vi "ScanDelay_FTIR_LineScanSpectroscopy.vi"() -> ()   [LabVIEW 2022 SP3]
uses:
  Control_scanDelayWorkflow.ctl
  Control_GetSpectrum_LineScanSpectroscopy.ctl
panel:
  out "Line done":bool
  out "Data needed at new point":bool
  out "Sample Spectra at all accumulations":dbl[][][][](array[numeric])
  in  "Next Point":bool
  out "Current point\nindex":i32=1
  in  "# of spatial points":i32=2
  in  "Spectra view":enum32{"Point Spectrum", "Linescan Spectrum"}(tab)
  out "Normalized spectrum (amplitude)":T1(graph)
  out "Normalized spectrum (phase)":T1(graph)
  in  "Norm. smoothing":dbl=6.0 min=0.0 max=100.0 step=0.1
  in  "Flip anyway":bool
  out "Replicated wavelength (nm)":dbl=7692.0
  in  "Piecewise flattening":i16 min=0 max=10 step=1
  in  "Sample atten.\npowers (%)":dbl[](array[numeric])=[100.0, 100.0, 50.0, 50.0, 50.0, 50.0, 50.0, 50.0]
  in  "Sample power (%)":dbl(slide)=90.90909090909092 min=0.0 max=100.0 scale=0.0..100.0
  in  "Cyc. per intfg. (BB)":i32=30
  out "Attenuation factor":dbl=0.9090909090909092
  out "Replication wavelengths":dbl[](array[numeric])=[15300.0, 15300.0, 14800.0, 14800.0, 14500.0, 14500.0, 14100.0, 14100.0, 13700.0, 13333.0, 12500.0, 11765.0, 11111.0, 10526.0, 10000.0, 9524.0, 9091.0, 8696.0, 8333.0, 8000.0, 7692.0, 7407.0, 7143.0, 6897.0, 6667.0, 6452.0, 6250.0, 6061.0, 5882.0, 5714.0, 5556.0, 5405.0, 5263.0, 5000.0, 0.0]
  out "Replicator wavelengths loaded":bool=TRUE
  in  "Replic. path":path=path "C:/Users/mnopl/Desktop/Software/mnOPSuite/PRISM/Alpha replicator tables/2022.12.1 - 550-2000cm-1_x30_ExtraLowEnergyLiam.txt"
  in  "Load replic. table":bool
  in  "BB attenuation\npowers (%)":dbl[](array[numeric])=[100.0, 50.0, 2.0, 2.0, 2.0, 2.0, 2.0, 2.0]
  in  "Attenuation\nenergies (cm-1)":dbl[](array[numeric])=[500.0, 750.0, 1000.0, 1200.0, 1550.0, 1650.0, 1800.0, 2000.0]
  in  "BB power (%)":dbl(slide)=96.96969696969697 min=0.0 max=100.0 scale=0.0..100.0
  in  "Power threshold":dbl(slide)=343.04692863149205 scale=10.0..1000.0
  in  "Update alignment":bool
  in  "Bright beam: alignment delay":i32=-12
  in  "Norm. phase offset":dbl
  in  "Bright beam: physical channels (inputV, ScanDelay X)":tag="Dev1/ai2,Dev1/ai3"
  in  "Sample: physical channels (inputV, ScanDelay X)":tag="Dev1/ai2,Dev1/ai3"
  in  "Sample: alignment delay":i32=-12
  in  "Path to save\nnormalized spectrum":path=path "D:/Dropbox/Data/Park-SNOM/2022.07.19 - Liam - Strained STO/12_7 Measurements/STO_NormTo_Au_S2.txt"
  in  "Save normalized\nspectrum":bool
  in  "Optimize\ninterferogram\nalignment":bool
  in  "Toggle BB\nmirror\nUp / Down":bool=TRUE
  in  "Realign phase":bool=TRUE
  in  "Level phase":bool=TRUE
  in  "Pause\nacquisition":bool
  in  "Replicate\nfrom #":i8 min=0
  in  "Envelope width":dbl(slide)=1.6893939393939394 scale=0.25..4.0
  in  "BB-reference spectrum":bool
  in  "Acquire only\nBB 100% curve":bool=TRUE
  in  "Toggle pause (ms)":dbl=1000.0
  out "BB-referenced spectrum (phase)":T1(graph)
  out "BB-referenced spectrum (amplitude)":T2(graph)
  out "Reference BB spectra":dbl[][](array[numeric])
  out "Reference spectra":dbl[][](array[numeric])
  out "Latest alpha cmd":string="@mir setpump 90.9"
  in  "Replicate\nalpha on\naccumulation":bool
  out "# Accumulated":i32=2
  in  "# of Accumulations":i32=2
  in  "Cancel\nacquisition":bool
  out "Toggle position":i32=2
  out "Spectrum stored":bool=TRUE
  out "Reference stored":bool
  in  "Store as reference":bool
  out "Python alpha rep path":path=path "C:/Users/mnopl/Desktop/software/mnOPSuite/PRISM/python/alpha.py"
  out "Activity status":string="Awaiting command"
  out "Acquisition status":string="Ready to acquire spectrum"
  in  "Path to save spectrum":path=path "D:/Dropbox/Data/Park-SNOM/2022.07.19 - Liam - Strained STO/11_30 Measurements/Spectra/S2_AuRef12_9.txt"
  in  "Load reference":bool
  in  "Path to load reference":path=path "D:/Dropbox/Data/Park-SNOM/2022.07.19 - Liam - Strained STO/12_7 Measurements/STO_undeformed_S2.txt"
  in  "Path to load spectrum":path=path "D:/Dropbox/Data/Park-SNOM/2022.07.19 - Liam - Strained STO/12_7 Measurements/STO_undeformed_S2.txt"
  in  "Apply spectral\nenvelope":bool=TRUE
  out "Binned interferogram":cluster{"X":dbl, "Y":dbl}[](graph)
  out "Sample BB Spectra":dbl[][](array[numeric])
  out "Python error: spectrum acquisition":errorcluster
  out "Python scandelay path":path=path "C:/Users/mnopl/Desktop/software/mnOPSuite/PRISM/python/scandelay_FTIR.py"
  in  "Time per\nacquisition (s)":dbl=0.18
  in  "Sampling rate":dbl=250000.0
  in  "Delay calibratior\nfactor (ps/V)":dbl=-2.432 format="%_6g"
  in  "Cyc. / intfg.\n(sample)":i32=30
  out "Accumulated spectrum (amplitude)":T1(graph)
  out "Acquisition cycle":dbl[][](graph)
  out "% averaged":dbl=100.0
  in  "Halt program":bool=TRUE
  out "Python error: activity loop":errorcluster
  in  "Load spectrum":bool
  in  "Save spectrum":bool
  in  "Normalize spectrum":bool
  in  "Acquire spectrum":bool
  # "ai6 (7ps): -2 to -5"
  # "ai2 (7ps): -12 to -15"
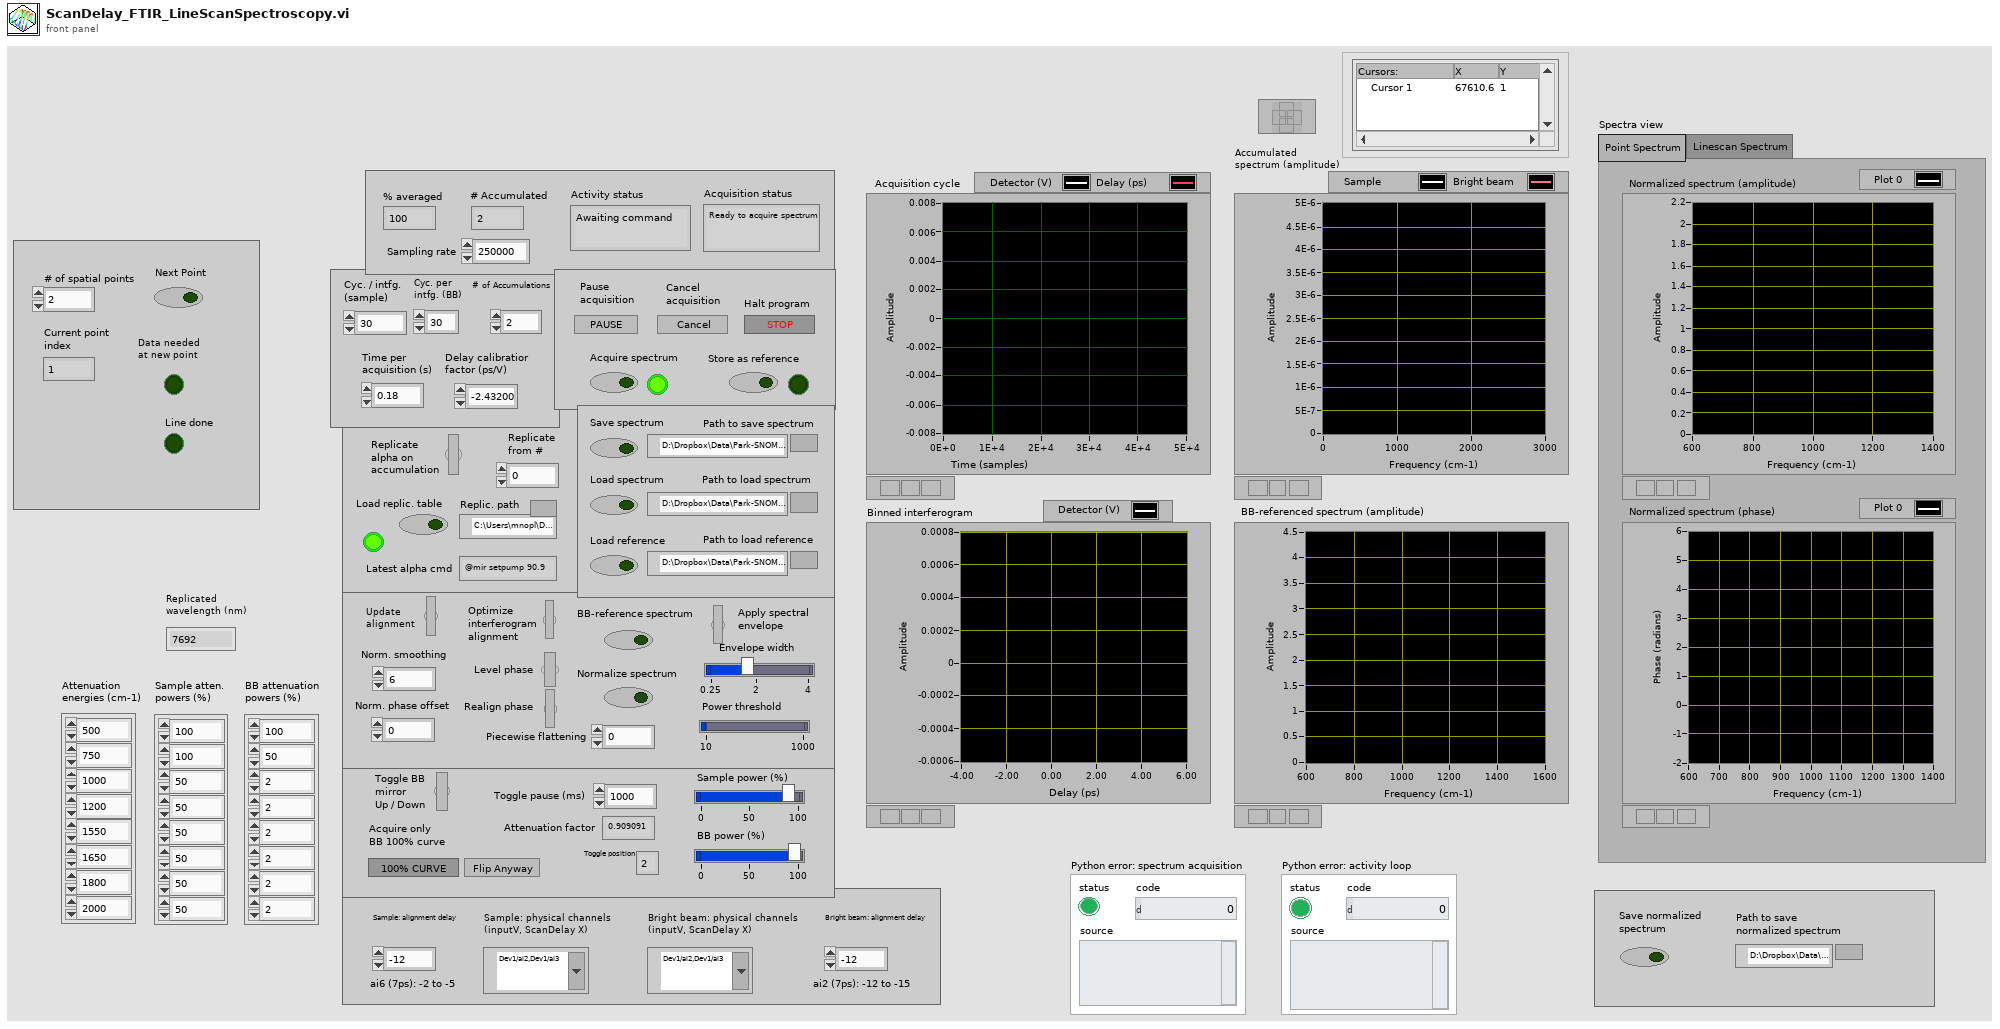
[diagram p1: front panel]
types:
  T1 = cluster{"Output spectrum":dbl[], "Output spectrum":dbl[]}
  T2 = cluster{"Sample Spectra":dbl[], "Sample Spectra":dbl[]}
  T3 = typedef "Control_scanDelayWorkflow.ctl" = enum16{"Initialize", "Sit Idle", "Load replicator table", "Flip BB", "Load Spectrum", "Store reference", "Save Spectrum", "Load reference", "Check Reference", "Check Spectrum", "BB reference spectrum", "Normalize Spectrum", "Save normalized spectrum", "Done"}
  T4 = typedef "imagedata.ctl" = cluster{"image type":i32, "image depth":i32, "image":u8[], "mask":u8[], "colors":u32[], "Rectangle":cluster{"left":i16, "top":i16, "right":i16, "bottom":i16}}
  T5 = typedef "Control_GetSpectrum_LineScanSpectroscopy.ctl" = enum16{"Initialize", "Replicate alpha", "Flip in BB", "Attenuate alpha", "Get Spectrum", "Accumulate BB spectrum", "Flip out BB", "Accumulate sample spectrum", "Await next point", "Assess accumulation", "Finalize", "Done"}
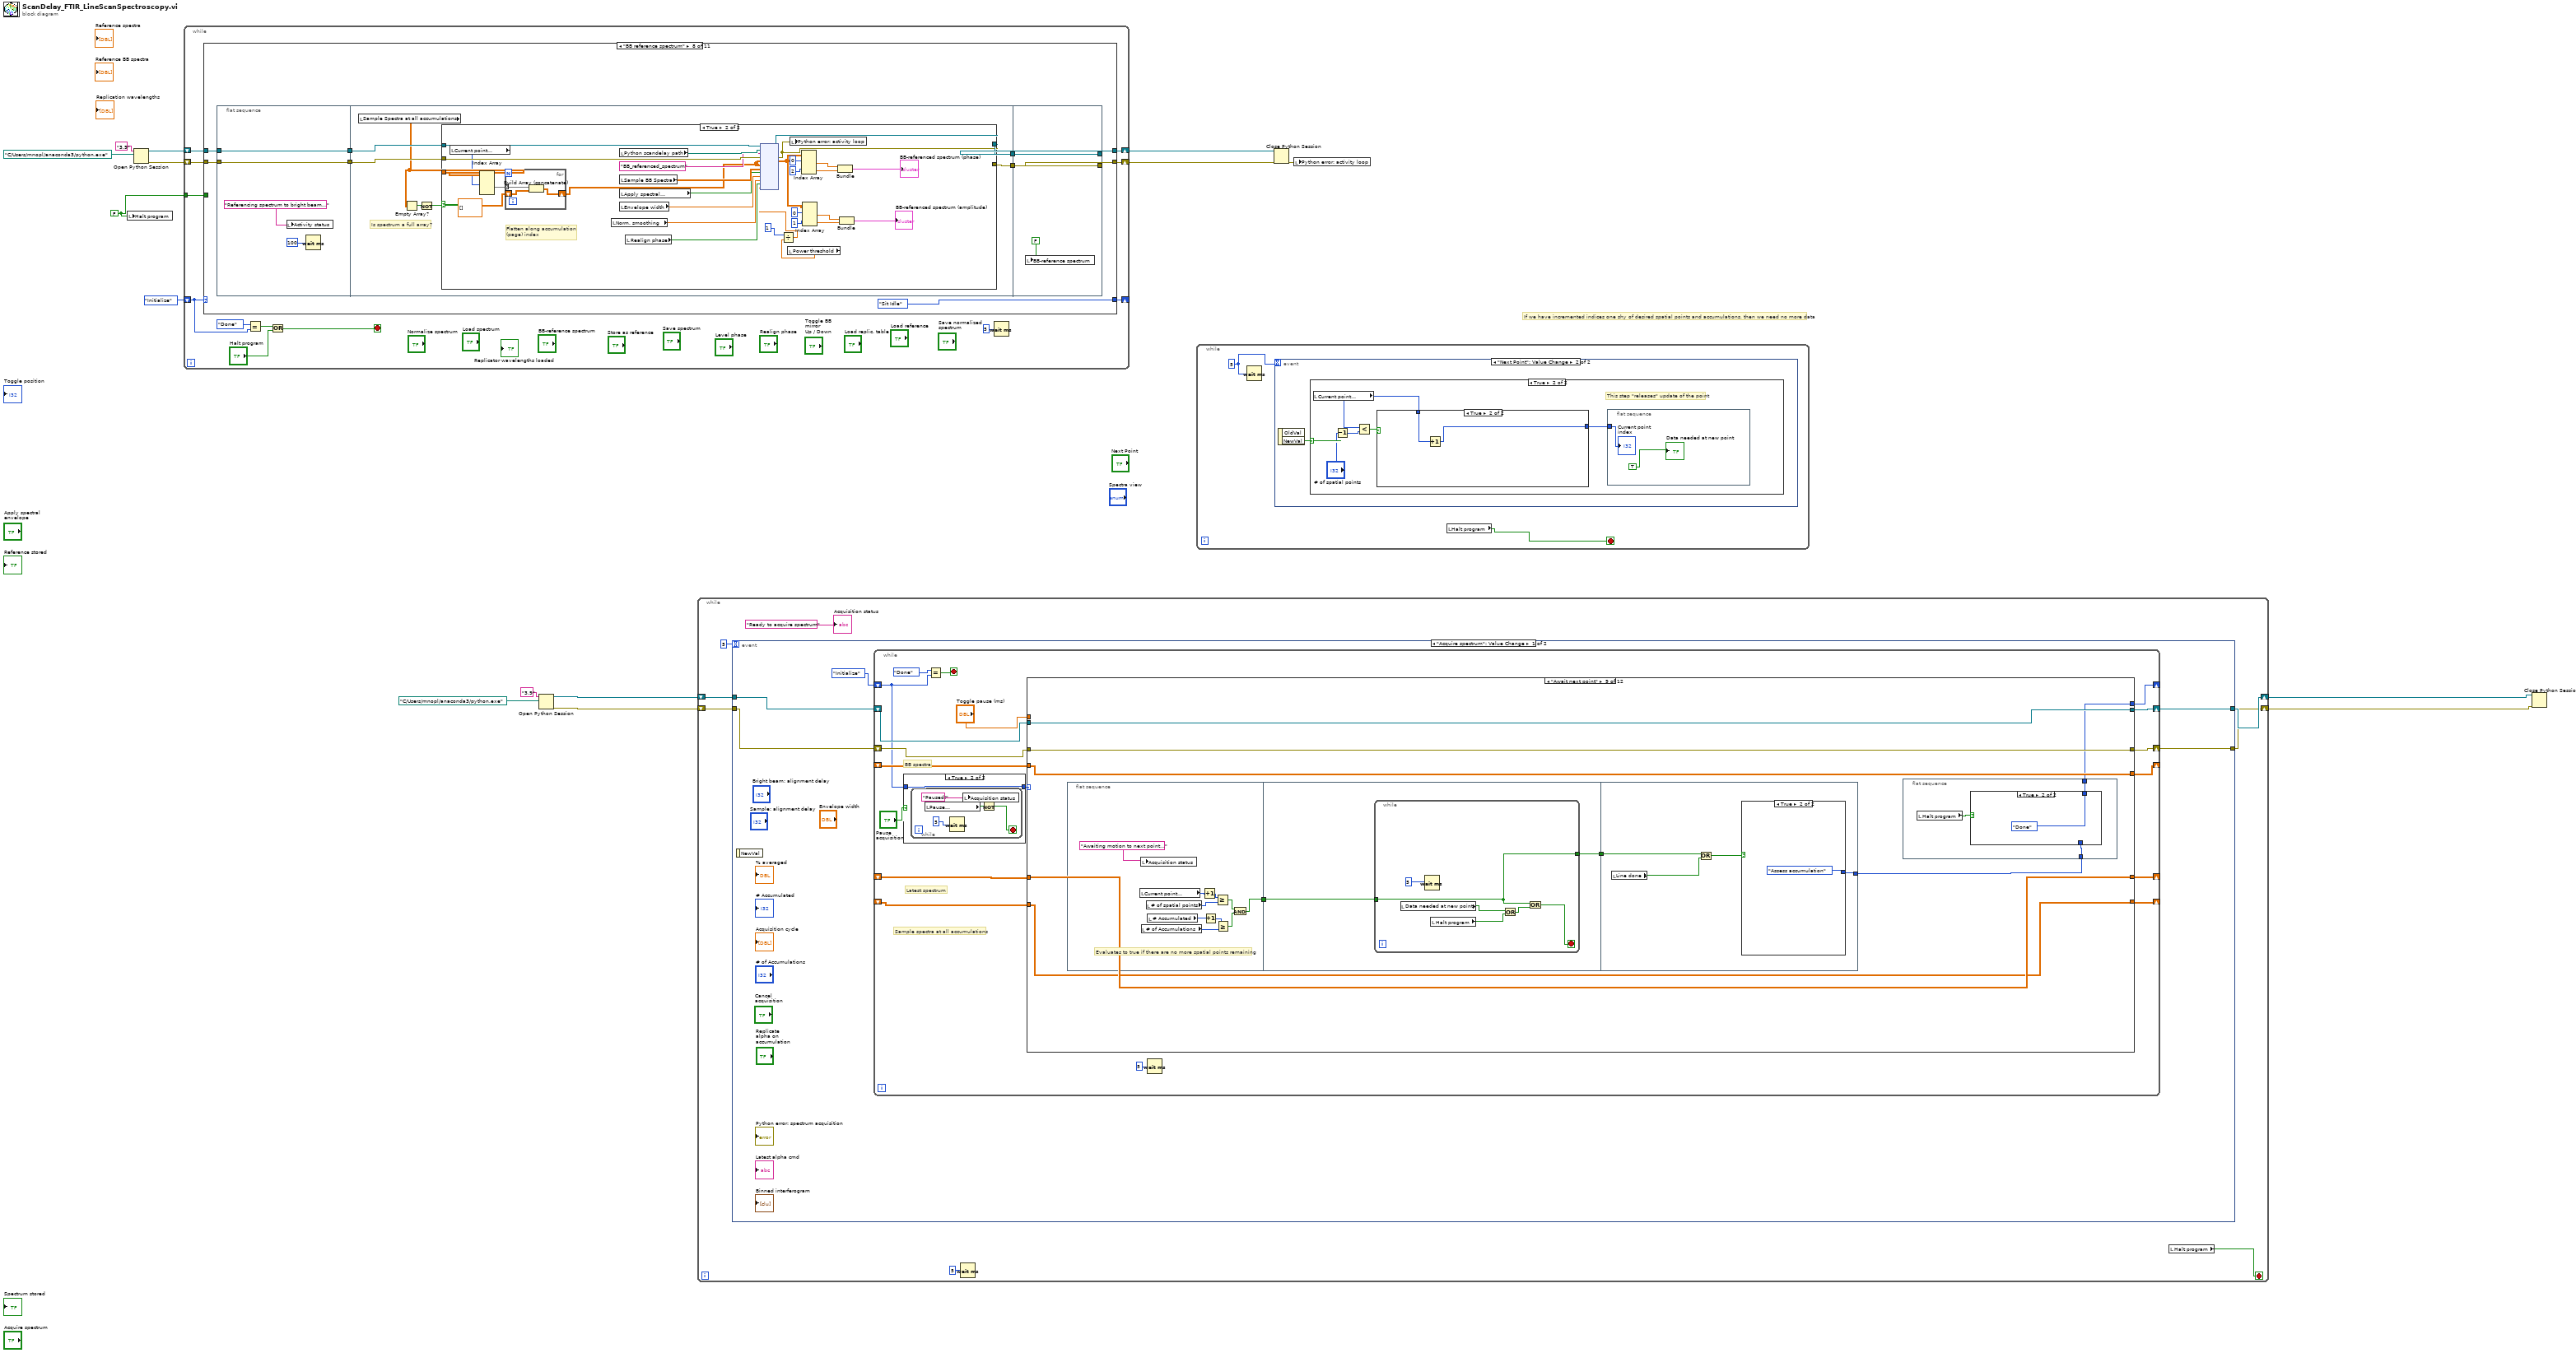
[diagram p0: block diagram]
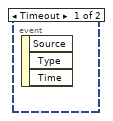
[diagram p2: hidden frame]
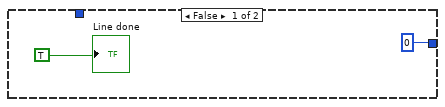
[diagram p4: hidden frame]
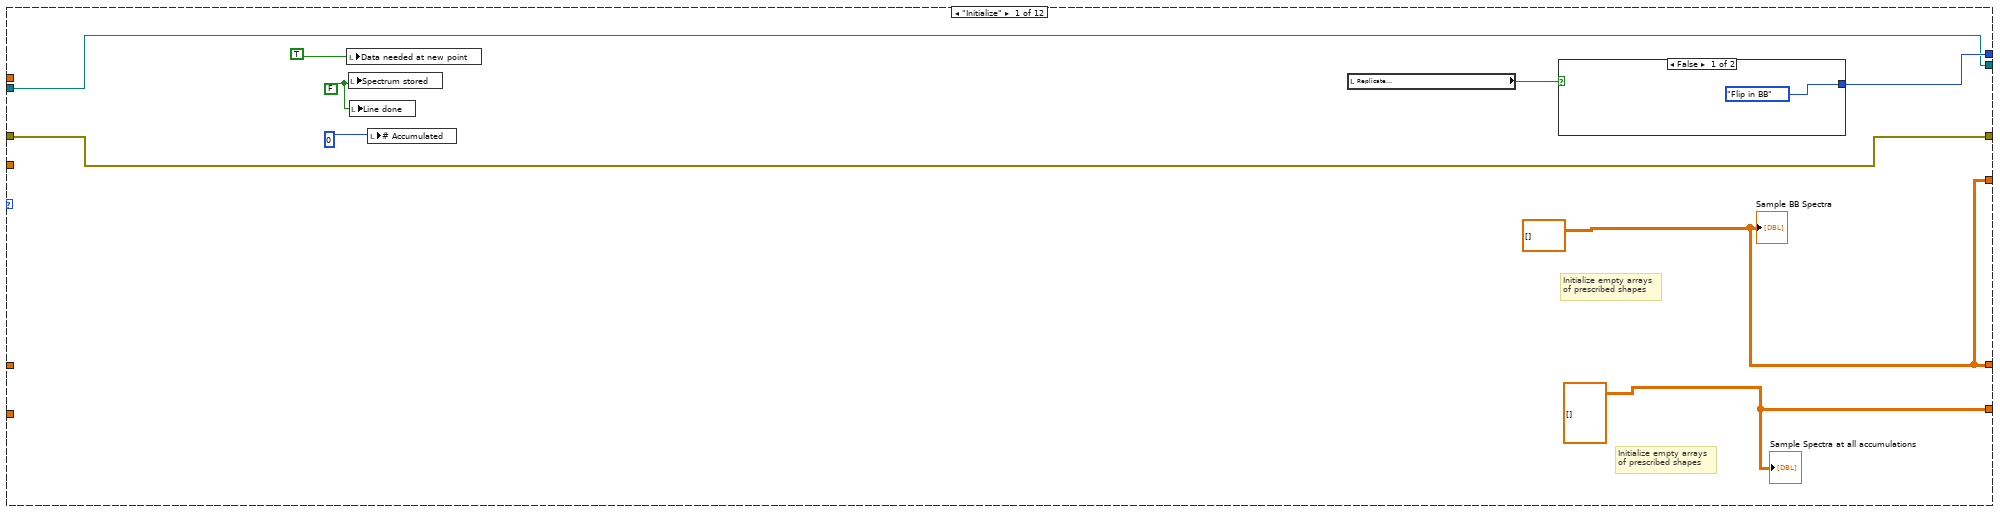
[diagram p6: hidden frame]
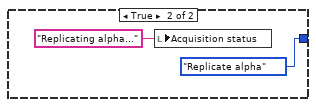
[diagram p7: hidden frame]
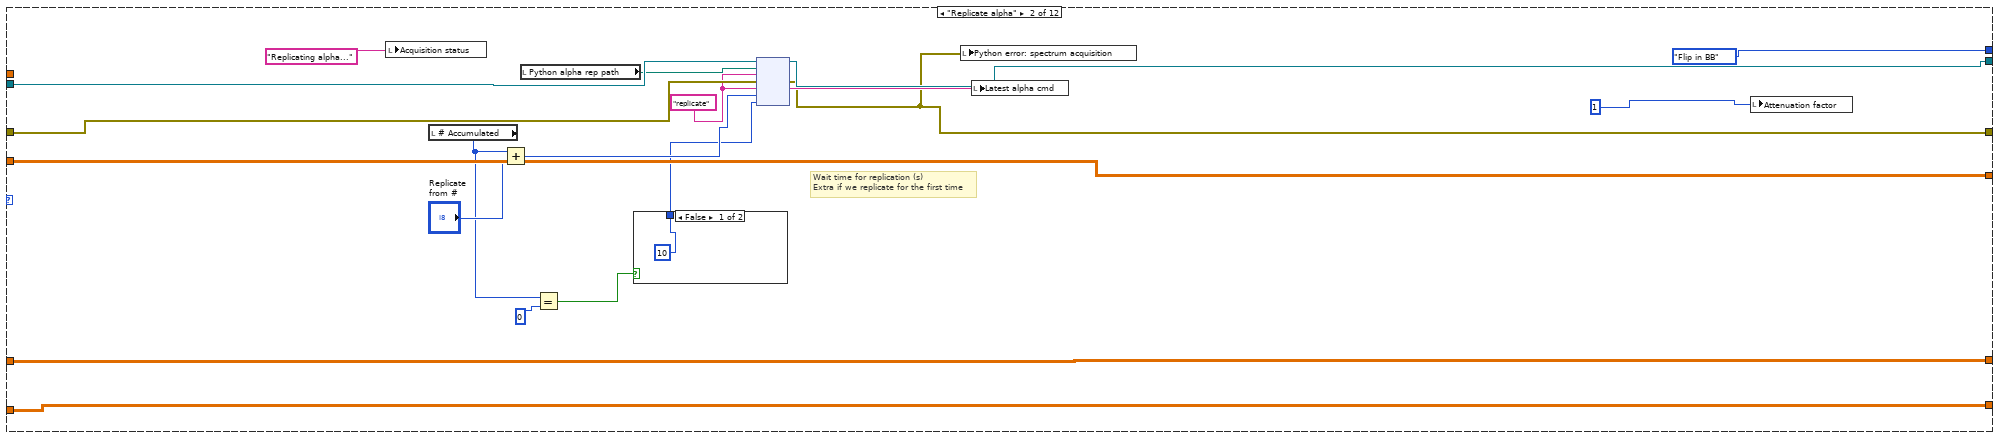
[diagram p8: hidden frame]
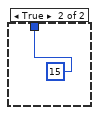
[diagram p9: hidden frame]
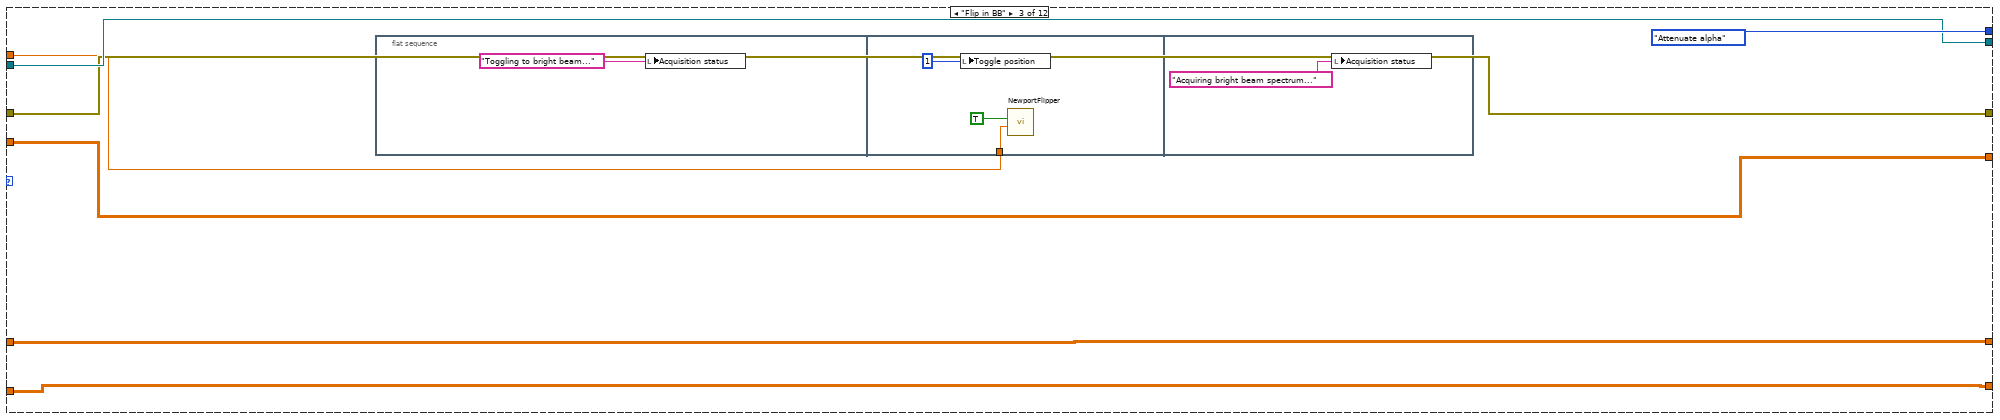
[diagram p10: hidden frame]
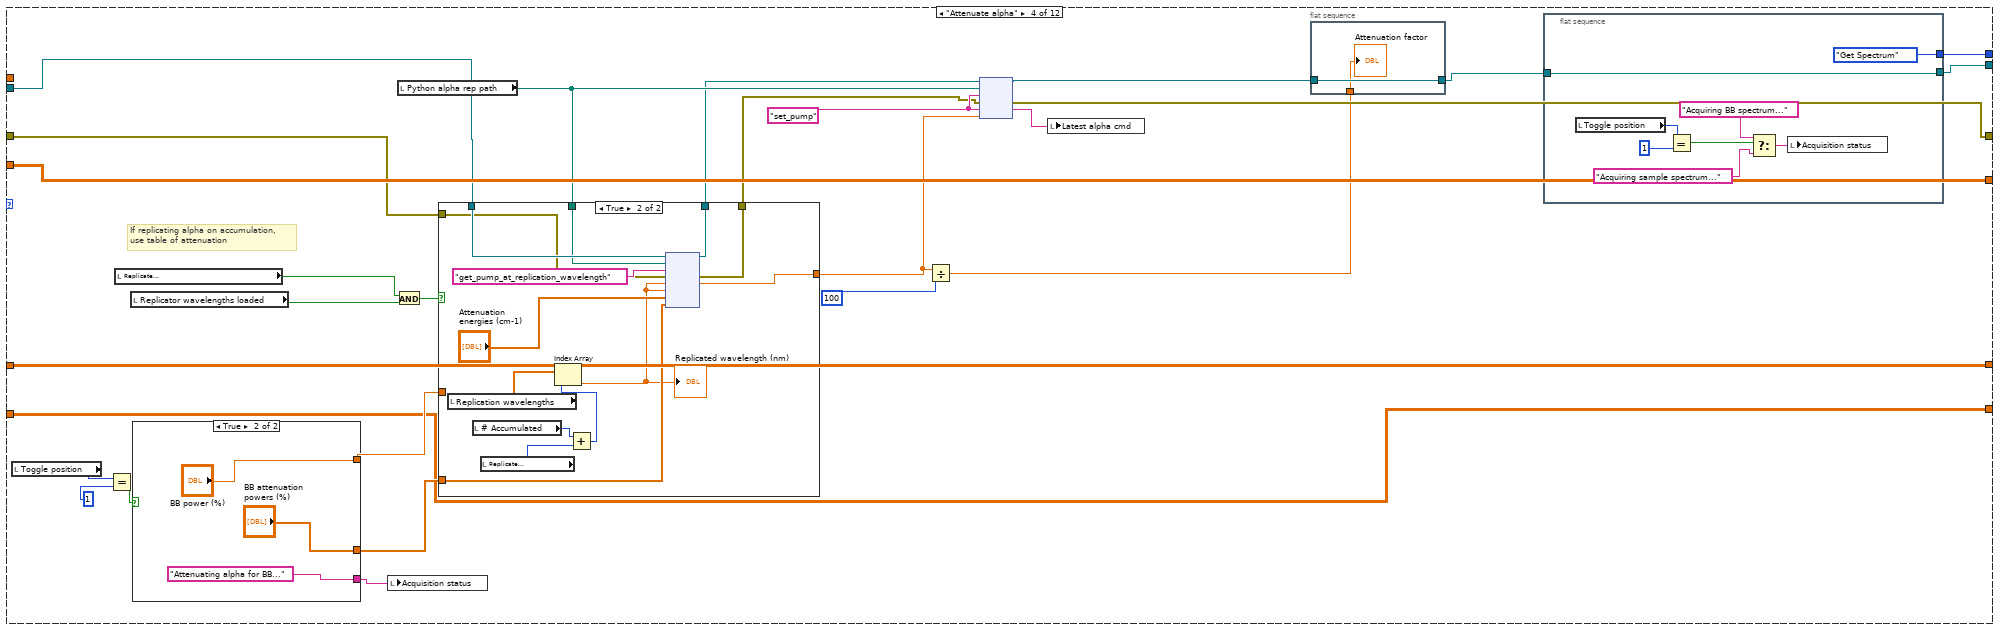
[diagram p11: hidden frame]
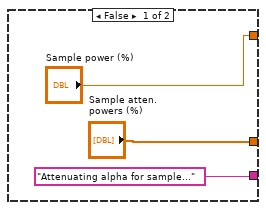
[diagram p12: hidden frame]
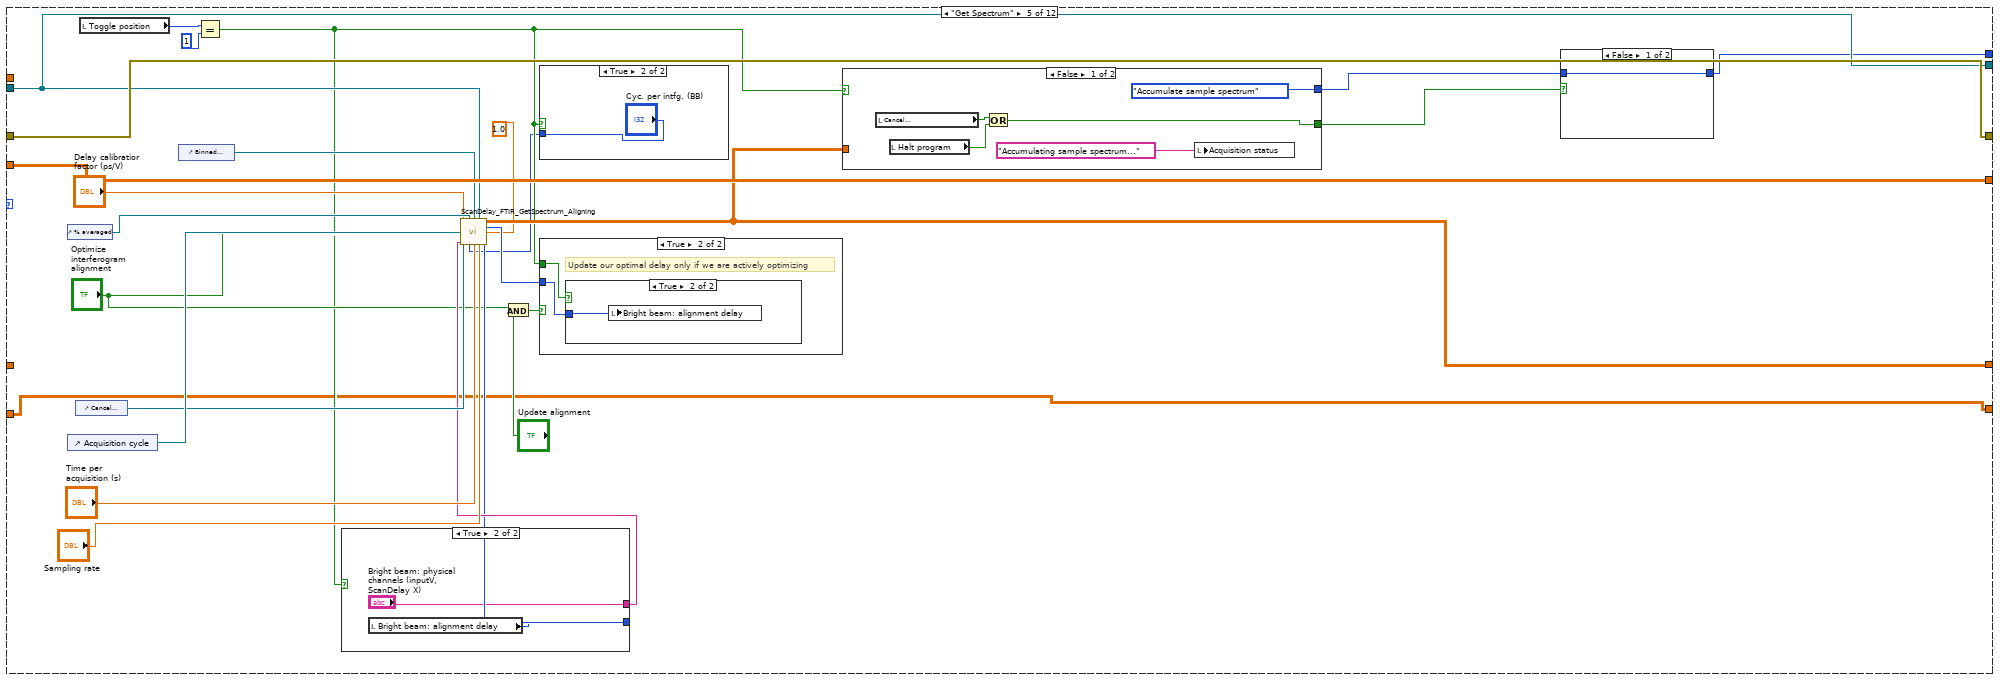
[diagram p14: hidden frame]
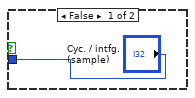
[diagram p15: hidden frame]
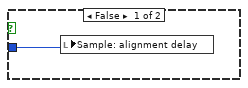
[diagram p17: hidden frame]
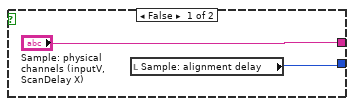
[diagram p18: hidden frame]
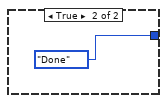
[diagram p19: hidden frame]
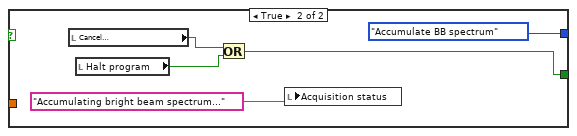
[diagram p20: hidden frame]
diagram:
  w1 = FALSE
  # "If we have incremented indices one shy of desired spatial points and accumulations, then we need no more data"
  n1 = local write "Halt program"(w1) -> ()
  n2 = Open Python Session(python version="3.9", python path=path "C:/Users/mnopl/anaconda3/python.exe") -> (session out=w11:refnum<k35>, error out=w10:errorcluster)  [unwired: 1 in]
  n3 = while {
    shift-right: [w20] -> _
    shift-left: Control_scanDelayWorkflow."Initialize" -> [w17]
    shift-right: [w26] -> w12
    shift-left: w10 -> [w18]
    shift-right: [w21] -> w13
    shift-left: w11 -> [w19]
    tunnel: w1 -> [w16]
    stop <- w24 stop-if-true
    n4 = case shown="\"BB reference spectrum\"" w17 {
      tunnel: [w31 w74 w93 w115 w136 w193 w216 w227 w280 w287 w331] -> w26
      tunnel: w19 -> [w32 w73 w92 w116 w139 w194 w217 w225 w281 w288 w332]
      tunnel: w18 -> [w31 w74 w93 w115 w138 w193 w216 w224 w280 w287 w331]
      tunnel: [w32 w73 w92 w116 w137 w194 w217 w226 w281 w288 w332] -> w21
      tunnel: [w30 Control_scanDelayWorkflow."Sit Idle" Control_scanDelayWorkflow."Sit Idle" Control_scanDelayWorkflow."Sit Idle" Control_scanDelayWorkflow."Sit Idle" Control_scanDelayWorkflow."Sit Idle" Control_scanDelayWorkflow."Sit Idle" Control_scanDelayWorkflow."Sit Idle" Control_scanDelayWorkflow."Sit Idle" Control_scanDelayWorkflow."Sit Idle" Control_scanDelayWorkflow."Sit Idle"] -> w20
      tunnel: w16 -> [_ _ _ _ _ _ w213 _ _ _ _]
      frame "Sit Idle", Default {
        n5 = event shown="[9] Timeout" {
          selector: _ -> [_ _ _ _ _ _ _ _ _ _]
          dyn-events: _ -> [_ _ _ _ _ _ _ _ _ _]
          timeout: 5 -> [_ _ _ _ _ _ _ _ _ w66]
          tunnel: [w33 w37 w44 Control_scanDelayWorkflow."Flip BB" w46 w50 w54 w58 w62 Control_scanDelayWorkflow."Sit Idle"] -> w30
          event "Normalize spectrum": Value Change {
            n6 = event-data() -> ("NewVal"=w34:bool)  [unwired: 1 in]
            n7 = Select(t=Control_scanDelayWorkflow."Normalize Spectrum", s=w34, f=Control_scanDelayWorkflow."Sit Idle") -> (s? t:f=w33:T3)
          }
          event "Store as reference": Value Change {
            n8 = event-data() -> ("NewVal"=w40:bool)  [unwired: 1 in]
            n9 = Select(t=Control_scanDelayWorkflow."Store reference", s=w40, f=Control_scanDelayWorkflow."Sit Idle") -> (s? t:f=w37:T3)
          }
          event "BB-reference spectrum": Value Change {
            n10 = event-data() -> ("NewVal"=w42:bool)  [unwired: 1 in]
            n11 = Select(t=Control_scanDelayWorkflow."BB reference spectrum", s=w42, f=Control_scanDelayWorkflow."Sit Idle") -> (s? t:f=w44:T3)
          }
          event "Toggle BB\nmirror\nUp / Down": Value Change {
            n12 = event-data() -> ()  [unwired: 1 in, 1 out]
          }
          event "Save normalized\nspectrum": Value Change {
            n13 = event-data() -> ("NewVal"=w47:bool)  [unwired: 1 in]
            n14 = Select(t=Control_scanDelayWorkflow."Save normalized spectrum", s=w47, f=Control_scanDelayWorkflow."Sit Idle") -> (s? t:f=w46:T3)
          }
          event "Load replic. table": Value Change {
            n15 = event-data() -> ("NewVal"=w53:bool)  [unwired: 1 in]
            n16 = Select(t=Control_scanDelayWorkflow."Load replicator table", s=w53, f=Control_scanDelayWorkflow."Sit Idle") -> (s? t:f=w50:T3)
          }
          event "Save spectrum": Value Change {
            n17 = event-data() -> ("NewVal"=w55:bool)  [unwired: 1 in]
            n18 = Select(t=Control_scanDelayWorkflow."Save Spectrum", s=w55, f=Control_scanDelayWorkflow."Sit Idle") -> (s? t:f=w54:T3)
          }
          event "Load reference": Value Change {
            n19 = event-data() -> ("NewVal"=w61:bool)  [unwired: 1 in]
            n20 = Select(t=Control_scanDelayWorkflow."Load reference", s=w61, f=Control_scanDelayWorkflow."Sit Idle") -> (s? t:f=w58:T3)
          }
          event "Load spectrum": Value Change {
            n21 = event-data() -> ("NewVal"=w63:bool)  [unwired: 1 in]
            n22 = Select(t=Control_scanDelayWorkflow."Load Spectrum", s=w63, f=Control_scanDelayWorkflow."Sit Idle") -> (s? t:f=w62:T3)
          }
          event Timeout {
            n23 = event-data() -> ()  [unwired: 1 in, 2 out]
            n24 = Wait (ms)(milliseconds to wait=w66) -> ()  [unwired: 1 out]
          }
        }
        "Activity status" <- "Awaiting command"
      }
      frame "Store reference" {
        # "Is spectrum a full array?"
        n25 = local read "Sample Spectra at all accumulations"() -> (w69:dbl[][][][])
        n26 = local read "Sample BB Spectra"() -> (w68:dbl[][])
        n27 = Empty Array?(array=w69) -> (empty?=w71:bool)
        n28 = Not(x=w71) -> (.not. x?=w70:bool)
        n29 = case shown="True" w70 {
          tunnel: w69 -> [_ w79]
          tunnel: w68 -> [_ w81]
          frame False {
            n30 = Wait (ms)(milliseconds to wait=1000) -> ()  [unwired: 1 out]
            n31 = local write "Activity status"("Error: Spectrum is empty!") -> ()
          }
          frame True {
            # "Flatten along accumulation\n(page) index"
            n32 = local read "Current point\nindex"() -> (w77:i32)
            n33 = Index Array(array=w79, index (dim 1)=w77) -> (element=w80:dbl[][][])  [unwired: 3 in]
            n34 = for {
              tunnel: w80 -> [w87] mode=indexing
              shift-right: [w86] -> w78
              shift-left: _ -> [w85]
              n35 = Build Array (concatenate)(w87, w85) -> (w86:dbl[][])
            }
            n36 = local write "Reference BB spectra"(w81) -> ()
            n37 = local write "Reference spectra"(w78) -> ()
            n38 = local write "Reference stored"(TRUE) -> ()
            n39 = Wait (ms)(milliseconds to wait=1000) -> ()  [unwired: 1 out]
            n40 = local write "Activity status"("Storing reference!") -> ()
          }
        }
      }
      frame "Save Spectrum" {
        # "Is spectrum a full array?"
        n41 = local read "Sample Spectra at all accumulations"() -> (w89:dbl[][][][])
        n42 = Empty Array?(array=w89) -> (empty?=w90:bool)
        n43 = Not(x=w90) -> (.not. x?=w88:bool)
        n44 = case shown="True" w88 {
          tunnel: w89 -> [_ w96]
          frame False {
            n45 = flat-sequence {
              frame #0 {
                n46 = local write "Activity status"("Error:  Spectrum is empty, cannot save!") -> ()
              }
              frame #1 {
                n47 = Wait (ms)(milliseconds to wait=1000) -> ()  [unwired: 1 out]
              }
            }
          }
          frame True {
            n48 = flat-sequence {
              tunnel: w96 -> [w97]
              frame #0 {
                w103 = "%g"
                n49 = Path To String(path="Path to save spectrum") -> (string=w106:string)
                n50 = local read "Sample BB Spectra"() -> (w98:dbl[][])
                n51 = Search and Replace String(input string=w106, search string="(.txt)*$", replace string=".txt") -> (result string=w110:string)  [unwired: 5 in, 3 out]
                n52 = Search and Replace String(input string=w110, search string=".txt$", replace string="_BB.txt") -> (result string=w109:string)  [unwired: 5 in, 3 out]
                n53 = String To Path(string=w110) -> (path=w107:path)
                n54 = Array To Spreadsheet String(array=w97, 3:w103) -> (spreadsheet string=w104:string)  [unwired: 1 in]
                n55 = Array To Spreadsheet String(array=w98, 3:w103) -> (spreadsheet string=w111:string)  [unwired: 1 in]
                n56 = String To Path(string=w109) -> (path=w108:path)
                n57 = Write to Text File(file (use dialog)=w107, text=w104) -> ()  [unwired: 2 in, 3 out]
                n58 = Write to Text File(file (use dialog)=w108, text=w111) -> ()  [unwired: 2 in, 3 out]
              }
              frame #1 {
                n59 = local write "Activity status"("Successfully saved spectrum!") -> ()
                n60 = Wait (ms)(milliseconds to wait=1000) -> ()  [unwired: 1 out]
              }
            }
          }
        }
      }
      frame "Load reference" {
        n61 = flat-sequence {
          frame #0 {
            w121 = "%g"
            n62 = Path To String(path="Path to load reference") -> (string=w117:string)
            n63 = Search and Replace String(input string=w117, search string=".txt$", replace string="_BB.txt") -> (result string=w119:string)  [unwired: 5 in, 3 out]
            n64 = Read from Text File(file (use dialog)="Path to load reference") -> (text=w122:string)  [unwired: 3 in, 3 out]
            n65 = String To Path(string=w119) -> (path=w126:path)
            n66 = Spreadsheet String To Array(format string=w121, spreadsheet string=w122) -> (array=w123:dbl[][])  [unwired: 2 in]
            n67 = Read from Text File(file (use dialog)=w126) -> (text=w125:string)  [unwired: 3 in, 3 out]
            n68 = local write "Reference spectra"(w123) -> ()
            n69 = Spreadsheet String To Array(format string=w121, spreadsheet string=w125) -> (array=w127:dbl[][])  [unwired: 2 in]
            n70 = local write "Reference BB spectra"(w127) -> ()
          }
          frame #1 {
            n71 = local write "Reference stored"(TRUE) -> ()
            n72 = Wait (ms)(milliseconds to wait=1000) -> ()  [unwired: 1 out]
            n73 = local write "Activity status"("Successfully loaded reference!") -> ()
          }
        }
      }
      frame "Normalize Spectrum" {
        n74 = local read "Reference stored"() -> (w133:bool)
        n75 = local read "Spectrum stored"() -> (w132:bool)
        n76 = And(x=w132, y=w133) -> (x .and. y?=w131:bool)
        n77 = flat-sequence {
          tunnel: w139 -> [w145]
          tunnel: w138 -> [w144]
          tunnel: [w143] -> w135
          tunnel: [w142] -> w134
          tunnel: w131 -> [w141]
          tunnel: [w190] -> w136
          tunnel: [w191] -> w137
          tunnel: w135 -> [w191]
          tunnel: w134 -> [w190]
          frame #0 {
            n78 = case shown="True" w141 {
              tunnel: w145 -> [w147 w184]
              tunnel: w144 -> [w146 w183]
              tunnel: [w147 w182] -> w143
              tunnel: [w146 w166] -> w142
              frame False {
                n79 = Wait (ms)(milliseconds to wait=1000) -> ()  [unwired: 1 out]
                n80 = local write "Activity status"("Error: Spectrum or reference is empty!") -> ()
              }
              frame True {
                # "Flatten along accumulation\n(page) index"
                n81 = local read "Sample Spectra at all accumulations"() -> (w152:dbl[][][][])
                n82 = local read "Current point\nindex"() -> (w151:i32)
                n83 = Index Array(array=w152, index (dim 1)=w151) -> (element=w153:dbl[][][])  [unwired: 3 in]
                n84 = for {
                  tunnel: w153 -> [w188] mode=indexing
                  shift-right: [w187] -> w150
                  shift-left: _ -> [w186]
                  n85 = Build Array (concatenate)(w188, w186) -> (w187:dbl[][])
                }
                n86 = Wait (ms)(milliseconds to wait=1000) -> ()  [unwired: 1 out]
                n87 = local read "Python scandelay path"() -> (w181:path)
                n88 = local read "Sample BB Spectra"() -> (w167:dbl[][])
                n89 = local read "Reference spectra"() -> (w165:dbl[][])
                n90 = local read "Reference BB spectra"() -> (w164:dbl[][])
                n91 = local read "Apply spectral\nenvelope"() -> (w163:bool)
                n92 = local read "Envelope width"() -> (w162:dbl)
                n93 = local read "Realign phase"() -> (w160:bool)
                n94 = local read "Level phase"() -> (w161:bool)
                n95 = local write "Activity status"("Normalizing spectrum!") -> ()
                n96 = Divide(x=1, y="Power threshold") -> (x/y=w155:dbl)
                n97 = node(w184, w181, "normalized_spectrum", w183, w150, w150, w167, w165, w164, w163, w162, w161, w160, "Norm. phase offset", "Norm. smoothing", w155, "Piecewise flattening") -> (w182:refnum<k35>, w166:errorcluster, w169:dbl[][])  [unwired: 12 in, 2 out]
                "Python error: activity loop" <- w166
                n98 = Index Array(array=w169, index (row) #1=0, index (row) #2=1) -> (element #1=w177:dbl[], element #2=w176:dbl[])  [unwired: 2 in]
                n99 = Index Array(array=w169, index (row) #1=0, index (row) #2=2) -> (element #1=w173:dbl[], element #2=w172:dbl[])  [unwired: 2 in]
                n100 = Bundle(w177, w176) -> (→"Normalized spectrum (amplitude)":cluster{dbl[], dbl[]})  [unwired: 1 in]
                n101 = Bundle(w173, w172) -> (→"Normalized spectrum (phase)":cluster{dbl[], dbl[]})  [unwired: 1 in]
              }
            }
          }
          frame #1 {
            n102 = local write "Normalize spectrum"(FALSE) -> ()
          }
        }
      }
      frame "Load Spectrum" {
        n103 = disable-structure shown="Disabled" {
          frame Disabled {
            n104 = flat-sequence {
              frame #0 {
                w202 = "%g"
                n105 = Path To String(path="Path to load spectrum") -> (string=w198:string)
                n106 = Search and Replace String(input string=w198, search string=".txt$", replace string="_BB.txt") -> (result string=w200:string)  [unwired: 5 in, 3 out]
                n107 = Read from Text File(file (use dialog)="Path to load spectrum") -> (text=w203:string)  [unwired: 3 in, 3 out]
                n108 = String To Path(string=w200) -> (path=w205:path)
                n109 = Spreadsheet String To Array(format string=w202, spreadsheet string=w203) -> (array=w196:dbl[][])  [unwired: 2 in]
                n110 = Read from Text File(file (use dialog)=w205) -> (text=w204:string)  [unwired: 3 in, 3 out]
                n111 = Spreadsheet String To Array(format string=w202, spreadsheet string=w204) -> (array=w195:dbl[][])  [unwired: 2 in]
                n112 = local write item#-1(w196) -> ()
                n113 = local write "Sample BB Spectra"(w195) -> ()
              }
              frame #1 {
                n114 = local write "Load spectrum"(FALSE) -> ()
                n115 = local write "Spectrum stored"(TRUE) -> ()
                n116 = local write "Activity status"("Successfully loaded spectrum!") -> ()
                n117 = Wait (ms)(milliseconds to wait=1000) -> ()  [unwired: 1 out]
              }
            }
          }
          frame Enabled {
          }
        }
      }
      frame "Initialize" {
        # "Fine so long as we've saved default values for \"replication wavelengths\""
        n118 = local write "Replicator wavelengths loaded"(TRUE) -> ()
        n119 = local write "Current point\nindex"(0) -> ()
        n120 = local write "Data needed at new point"(FALSE) -> ()
        n121 = local write "Reference stored"(w213) -> ()
        n122 = local write "Spectrum stored"(w213) -> ()
        n123 = local write "Acquire spectrum"(w213) -> ()
        "Python scandelay path" <- path "C:/Users/mnopl/Desktop/software/mnOPSuite/PRISM/python/scandelay_FTIR.py"
        "Python alpha rep path" <- path "C:/Users/mnopl/Desktop/software/mnOPSuite/PRISM/python/alpha.py"
      }
      frame "BB reference spectrum" {
        n124 = flat-sequence {
          tunnel: w224 -> [w230]
          tunnel: w225 -> [w231]
          tunnel: [w231] -> w220
          tunnel: [w230] -> w219
          tunnel: [w238] -> w222
          tunnel: [w237] -> w221
          tunnel: w220 -> [w236]
          tunnel: w219 -> [w235]
          tunnel: [w277] -> w226
          tunnel: [w278] -> w227
          tunnel: w222 -> [w278]
          tunnel: w221 -> [w277]
          frame #0 {
            n125 = local write "Activity status"("Referencing spectrum to bright beam...") -> ()
            n126 = Wait (ms)(milliseconds to wait=100) -> ()  [unwired: 1 out]
          }
          frame #1 {
            # "Is spectrum a full array?"
            n127 = local read "Sample Spectra at all accumulations"() -> (w232:dbl[][][][])
            n128 = Empty Array?(array=w232) -> (empty?=w234:bool)
            n129 = Not(x=w234) -> (.not. x?=w233:bool)
            n130 = case shown="True" w233 {
              tunnel: [w239 w255] -> w238
              tunnel: [w240 w256] -> w237
              tunnel: w236 -> [w240 w262]
              tunnel: w235 -> [w239 w261]
              tunnel: w232 -> [_ w247]
              frame False {
                n131 = Wait (ms)(milliseconds to wait=500) -> ()  [unwired: 1 out]
                n132 = local write "Activity status"("Error: Spectrum or reference is empty!") -> ()
              }
              frame True {
                # "Flatten along accumulation\n(page) index"
                n133 = local read "Current point\nindex"() -> (w246:i32)
                n134 = Index Array(array=w247, index (dim 1)=w246) -> (element=w245:dbl[][][])  [unwired: 3 in]
                n135 = for {
                  tunnel: w245 -> [w275] mode=indexing
                  shift-right: [w274] -> w244
                  shift-left: dbl[][] [] -> [w273]
                  n136 = Build Array (concatenate)(w275, w273) -> (w274:dbl[][])
                }
                n137 = local read "Norm. smoothing"() -> (w248:dbl)
                n138 = local read "Python scandelay path"() -> (w259:path)
                n139 = local read "Sample BB Spectra"() -> (w260:dbl[][])
                n140 = local read "Apply spectral\nenvelope"() -> (w254:bool)
                n141 = local read "Envelope width"() -> (w253:dbl)
                n142 = local read "Realign phase"() -> (w252:bool)
                n143 = local read "Power threshold"() -> (w250:dbl)
                n144 = Divide(x=1, y=w250) -> (x/y=w249:dbl)
                n145 = node(w262, w259, "BB_referenced_spectrum", w261, w244, w244, w260, w254, w253, w248, w252, w249) -> (w256:refnum<k35>, w255:errorcluster, w267:dbl[][])  [unwired: 7 in, 2 out]
                n146 = local write "Python error: activity loop"(w255) -> ()
                n147 = Index Array(array=w267, index (row) #1=0, index (row) #2=2) -> (element #1=w270:dbl[], element #2=w269:dbl[])  [unwired: 2 in]
                n148 = Index Array(array=w267, index (row) #1=0, index (row) #2=1) -> (element #1=w272:dbl[], element #2=w271:dbl[])  [unwired: 2 in]
                n149 = Bundle(w270, w269) -> (→"BB-referenced spectrum (phase)":cluster{dbl[], dbl[]})  [unwired: 1 in]
                n150 = Bundle(w272, w271) -> (→"BB-referenced spectrum (amplitude)":cluster{dbl[], dbl[]})  [unwired: 1 in]
              }
            }
          }
          frame #2 {
            n151 = local write "BB-reference spectrum"(FALSE) -> ()
          }
        }
      }
      frame "Flip BB" {
        n152 = local read "Toggle BB\nmirror\nUp / Down"() -> (w283:bool)
        n153 = local read "Toggle pause (ms)"() -> (w279:dbl)
        n154 = call "NewportFlipper.vi"("Settle time (ms)"=w279, "Up/Down"=w283) -> ()  [unwired: 10 in]
      }
      frame "Save normalized spectrum" {
        n155 = flat-sequence {
          tunnel: [w302] -> w289
          tunnel: [w290] -> w284
          tunnel: w289 -> [w316]
          tunnel: [w313] -> w285
          tunnel: w284 -> [w313]
          tunnel: w285 -> [w325]
          frame #0 {
            w307 = "%g"
            n156 = Path To String(path="Path to save\nnormalized spectrum") -> (string=w302:string)
            n157 = property on="Normalized spectrum (phase)" class="XYGraph (strict)"() -> ("Value"=w292:T1)  [unwired: 2 in, 2 out]
            n158 = property on="Normalized spectrum (amplitude)" class="XYGraph (strict)"() -> ("Value"=w300:T1)  [unwired: 2 in, 2 out]
            n159 = Unbundle(w300) -> ("Output spectrum"=w299:dbl[], "Output spectrum"=w298:dbl[])
            n160 = Unbundle(w292) -> ("Output spectrum"=w295:dbl[], "Output spectrum"=w294:dbl[])
            n161 = Build Array(w299, w298) -> (w297:dbl[][])
            n162 = Build Array(w295, w294) -> (w293:dbl[][])
            n163 = Search and Replace String(input string=w302, search string="(.txt)$", replace string="_normalized_phase.txt") -> (result string=w311:string)  [unwired: 5 in, 3 out]
            n164 = Search and Replace String(input string=w302, search string="(.txt)*$", replace string="_normalized_amplitude.txt") -> (result string=w290:string)  [unwired: 5 in, 3 out]
            n165 = Transpose 2D Array(2D array=w297) -> (transposed array=w296:dbl[][])
            n166 = Transpose 2D Array(2D array=w293) -> (transposed array=w291:dbl[][])
            n167 = Array To Spreadsheet String(array=w296, 3:w307) -> (spreadsheet string=w312:string)  [unwired: 1 in]
            n168 = Array To Spreadsheet String(array=w291, 3:w307) -> (spreadsheet string=w308:string)  [unwired: 1 in]
            n169 = String To Path(string=w311) -> (path=w310:path)
            n170 = String To Path(string=w290) -> (path=w309:path)
            n171 = Write to Text File(file (use dialog)=w310, text=w312) -> ()  [unwired: 2 in, 3 out]
            n172 = Write to Text File(file (use dialog)=w309, text=w308) -> ()  [unwired: 2 in, 3 out]
          }
          frame #1 {
            n173 = invoke on="Normalized spectrum (amplitude)" class="XYGraph (strict)" method="Get Image"() -> ("image data"=w315:T4)  [unwired: 6 in, 5 out]
            n174 = Search and Replace String(input string=w316, search string="(.txt)$", replace string="_normalized_amplitude.png") -> (result string=w322:string)  [unwired: 5 in, 3 out]
            n175 = String To Path(string=w322) -> (path=w321:path)
            n176 = call <vilib>:"Write PNG File.vi"("image data"=w315, "path to PNG file"=w321) -> ()  [unwired: 8 in, 2 out]
            n177 = invoke on="Normalized spectrum (phase)" class="XYGraph (strict)" method="Get Image"() -> ("image data"=w314:T4)  [unwired: 6 in, 5 out]
            n178 = Search and Replace String(input string=w316, search string="(.txt)$", replace string="_normalized_phase.png") -> (result string=w318:string)  [unwired: 5 in, 3 out]
            n179 = String To Path(string=w318) -> (path=w317:path)
            n180 = call <vilib>:"Write PNG File.vi"("image data"=w314, "path to PNG file"=w317) -> ()  [unwired: 8 in, 2 out]
          }
          frame #2 {
            n181 = local write "Save normalized\nspectrum"(FALSE) -> ()
            n182 = Concatenate Strings("Spectrum successfully saved to:" ("message"), "\r", w325) -> (w328:string)
            n183 = One Button Dialog(message=w328, button name ("OK")="OK") -> ()  [unwired: 1 out]
          }
        }
      }
      frame "Load replicator table" {
        n184 = flat-sequence {
          frame #0 {
            # "A leading whitespace in replication table requires skipping an extra column"
            n185 = Read from Text File(file (use dialog)="Replic. path") -> (text=w340:string)  [unwired: 3 in, 3 out]
            n186 = Spreadsheet String To Array(delimiter (Tab)=" ", format string="%g", spreadsheet string=w340) -> (array=w337:dbl[][])  [unwired: 1 in]
            n187 = Index Array(array=w337, index (col)=4) -> (element=w335:dbl[])  [unwired: 1 in]
            n188 = local write "Replication wavelengths"(w335) -> ()
          }
          frame #1 {
            n189 = local write "Load replic. table"(FALSE) -> ()
            n190 = local write "Replicator wavelengths loaded"(TRUE) -> ()
            n191 = Wait (ms)(milliseconds to wait=1000) -> ()  [unwired: 1 out]
            n192 = local write "Activity status"("Successfully loaded replication wavelengths!") -> ()
          }
        }
      }
    }
    n193 = Equal?(x=Control_scanDelayWorkflow."Done", y=w17) -> (x = y?=w22:bool)
    n194 = Or(x=w22, y="Halt program") -> (x .or. y?=w24:bool)
    n195 = Wait (ms)(milliseconds to wait=5) -> ()  [unwired: 1 out]
  }
  n196 = Open Python Session(python version="3.9", python path=path "C:/Users/mnopl/anaconda3/python.exe") -> (session out=w5:refnum<k35>, error out=w4:errorcluster)  [unwired: 1 in]
  n197 = while {
    shift-right: [w345] -> w2
    shift-left: w4 -> [w347]
    shift-right: [w346] -> w3
    shift-left: w5 -> [w348]
    stop <- w352 stop-if-true
    n198 = event shown="[0] \"Acquire spectrum\": Value Change" {
      selector: _ -> [_ _]
      dyn-events: _ -> [_ _]
      timeout: 5 -> [_ w711]
      tunnel: w348 -> [w356 w710]
      tunnel: w347 -> [w355 w709]
      tunnel: [w354 w710] -> w346
      tunnel: [w353 w709] -> w345
      event "Acquire spectrum": Value Change {
        n199 = event-data() -> ()  [unwired: 1 in, 1 out]
        n200 = while {
          shift-right: [w374] -> _
          shift-left: _ -> [w373]
          shift-right: [w372] -> _
          shift-left: Control_GetSpectrum_LineScanSpectroscopy."Initialize" -> [w362]
          shift-right: [w369] -> w353
          shift-left: w355 -> [w370]
          shift-right: [w368] -> w354
          shift-left: w356 -> [w371]
          shift-right: [w367] -> _
          shift-left: _ -> [w365]
          shift-right: [w359] -> _
          shift-left: _ -> [w358]
          stop <- w361 stop-if-true
          # "Sample spectra at all accumulations"
          # "BB spectra"
          # "Latest spectrum"
          n201 = case shown="True" "Pause\nacquisition" {
            tunnel: w362 -> [w376 w377]
            tunnel: [w376 w377] -> w360
            frame False {
            }
            frame True {
              n202 = while {
                stop <- w381 stop-if-true
                n203 = local read "Pause\nacquisition"() -> (w380:bool)
                n204 = Wait (ms)(milliseconds to wait=5) -> ()  [unwired: 1 out]
                n205 = local write "Acquisition status"("Paused!") -> ()
                n206 = Not(x=w380) -> (.not. x?=w381:bool)
              }
            }
          }
          n207 = Equal?(x=Control_GetSpectrum_LineScanSpectroscopy."Done", y=w362) -> (x = y?=w361:bool)
          n208 = case shown="\"Await next point\"" w360 {
            tunnel: [w383 w412 w418 w452 w511 w553 w571 w602 w639 w673 w697 w706] -> w374
            tunnel: w373 -> [_ w412 w418 w452 w511 w536 w571 w602 w639 w673 w697 w706]
            tunnel: [w390 Control_GetSpectrum_LineScanSpectroscopy."Flip in BB" Control_GetSpectrum_LineScanSpectroscopy."Attenuate alpha" w431 w498 w543 Control_GetSpectrum_LineScanSpectroscopy."Attenuate alpha" Control_GetSpectrum_LineScanSpectroscopy."Await next point" w636 w675 Control_GetSpectrum_LineScanSpectroscopy."Done" Control_GetSpectrum_LineScanSpectroscopy."Done"] -> w372
            tunnel: w371 -> [w387 w409 w420 w440 w508 w557 w570 w612 w641 w676 w699 w708]
            tunnel: w370 -> [w386 w408 w419 w444 w512 w556 w569 w611 w640 w677 w698 w707]
            tunnel: [w386 w403 w419 w451 w512 w547 w569 w603 w640 w677 w698 w707] -> w369
            tunnel: [w387 w404 w420 w429 w508 w555 w570 w610 w641 w676 w699 w708] -> w368
            tunnel: [w383 w402 w417 w453 w501 w548 w568 w591 w638 w674 w701 w705] -> w367
            tunnel: w365 -> [_ w402 w417 w453 _ w548 w568 w591 w638 w674 w701 w705]
            tunnel: "Toggle pause (ms)" -> [_ _ w416 _ _ _ w567 _ _ _ _ _]
            tunnel: [w385 w394 w415 w428 w487 w537 w566 w593 w637 w672 w695 w702] -> w359
            tunnel: w358 -> [_ w394 w415 w428 w487 w537 w566 w596 w637 w672 w695 w702]
            frame "Initialize" {
              w385 = dbl[][][][] []
              w384 = FALSE
              w383 = dbl[][] []
              # "Initialize empty arrays\nof prescribed shapes"
              # "Initialize empty arrays\nof prescribed shapes"
              n209 = local write "Data needed at new point"(TRUE) -> ()
              n210 = local write "Spectrum stored"(w384) -> ()
              n211 = local write "Line done"(w384) -> ()
              n212 = local write "# Accumulated"(0) -> ()
              n213 = local read "Replicate\nalpha on\naccumulation"() -> (w388:bool)
              n214 = case shown="False" w388 {
                tunnel: [Control_GetSpectrum_LineScanSpectroscopy."Flip in BB" Control_GetSpectrum_LineScanSpectroscopy."Replicate alpha"] -> w390
                frame False {
                }
                frame True {
                  n215 = local write "Acquisition status"("Replicating alpha...") -> ()
                }
              }
              "Sample BB Spectra" <- w383
              "Sample Spectra at all accumulations" <- w385
            }
            frame "Replicate alpha" {
              w406 = "replicate"
              # "Wait time for replication (s)\nExtra if we replicate for the first time"
              n216 = local write "Acquisition status"("Replicating alpha...") -> ()
              n217 = local read "# Accumulated"() -> (w398:i32)
              n218 = Add(x=w398, y="Replicate\nfrom #") -> (x+y=w400:i32)
              n219 = local read "Python alpha rep path"() -> (w407:path)
              n220 = Equal?(x=w398, y=0) -> (x = y?=w397:bool)
              n221 = case shown="False" w397 {
                tunnel: [10 15] -> w396
                frame False {
                }
                frame True {
                }
              }
              n222 = node(w409, w407, w406, w408, w406, w400, w396) -> (w404:refnum<k35>, w403:errorcluster, w405:string)  [unwired: 2 in, 2 out]
              n223 = local write "Python error: spectrum acquisition"(w403) -> ()
              n224 = local write "Latest alpha cmd"(w405) -> ()
              n225 = local write "Attenuation factor"(1) -> ()
            }
            frame "Flip in BB" {
              n226 = flat-sequence {
                tunnel: w416 -> [w423]
                frame #0 {
                  n227 = local write "Acquisition status"("Toggling to bright beam...") -> ()
                }
                frame #1 {
                  n228 = local write "Toggle position"(1) -> ()
                  n229 = call "NewportFlipper.vi"("Settle time (ms)"=w423, "Up/Down"=TRUE) -> ()  [unwired: 10 in]
                }
                frame #2 {
                  n230 = local write "Acquisition status"("Acquiring bright beam spectrum...") -> ()
                }
              }
            }
            frame "Attenuate alpha" {
              w450 = "set_pump"
              # "If replicating alpha on accumulation,\nuse table of attenuation"
              n231 = local read "Toggle position"() -> (w436:i32)
              n232 = Equal?(x=w436, y=1) -> (x = y?=w437:bool)
              n233 = local read "Replicate\nalpha on\naccumulation"() -> (w441:bool)
              n234 = local read "Replicator wavelengths loaded"() -> (w446:bool)
              n235 = case shown="True" w437 {
                tunnel: ["Sample power (%)" "BB power (%)"] -> w434
                tunnel: ["Sample atten.\npowers (%)" "BB attenuation\npowers (%)"] -> w433
                tunnel: ["Attenuating alpha for sample..." "Attenuating alpha for BB..."] -> w427
                frame False {
                }
                frame True {
                }
              }
              n236 = local write "Acquisition status"(w427) -> ()
              n237 = And(x=w441, y=w446) -> (x .and. y?=w447:bool)
              n238 = local read "Python alpha rep path"() -> (w445:path)
              n239 = case shown="True" w447 {
                tunnel: [w470 w475] -> w432
                tunnel: w440 -> [w472 w482]
                tunnel: w445 -> [_ w481]
                tunnel: w444 -> [w471 w479]
                tunnel: [w472 w478] -> w443
                tunnel: [w471 w477] -> w442
                tunnel: w434 -> [w470 _]
                tunnel: w433 -> [_ w474]
                frame False {
                }
                frame True {
                  n240 = local read "Replication wavelengths"() -> (w484:dbl[])
                  n241 = local read "# Accumulated"() -> (w485:i32)
                  n242 = local read "Replicate\nfrom #"() -> (w486:i8)
                  n243 = Add(x=w485, y=w486) -> (x+y=w483:i32)
                  n244 = Index Array(array=w484, index=w483) -> (element=w473:dbl)
                  "Replicated wavelength (nm)" <- w473
                  n245 = node(w482, w481, "get_pump_at_replication_wavelength", w479, w473, w473, "Attenuation\nenergies (cm-1)", w474) -> (w478:refnum<k35>, w477:errorcluster, w475:dbl)  [unwired: 3 in, 2 out]
                }
              }
              n246 = Divide(x=w432, y=100) -> (x/y=w438:dbl)
              n247 = node(w443, w445, w450, w442, w450, w432) -> (w439:refnum<k35>, w451:errorcluster, w449:string)  [unwired: 1 in, 2 out]
              n248 = local write "Latest alpha cmd"(w449) -> ()
              n249 = flat-sequence {
                tunnel: w439 -> [w469]
                tunnel: [w469] -> w430
                tunnel: w438 -> [w468]
                frame #0 {
                  "Attenuation factor" <- w468
                }
              }
              n250 = flat-sequence {
                tunnel: [Control_GetSpectrum_LineScanSpectroscopy."Get Spectrum"] -> w431
                tunnel: w430 -> [w460]
                tunnel: [w460] -> w429
                frame #0 {
                  n251 = local read "Toggle position"() -> (w458:i32)
                  n252 = Equal?(x=w458, y=1) -> (x = y?=w457:bool)
                  n253 = Select(t="Acquiring BB spectrum...", s=w457, f="Acquiring sample spectrum...") -> (s? t:f=w454:string)
                  n254 = local write "Acquisition status"(w454) -> ()
                }
              }
            }
            frame "Get Spectrum" {
              n255 = control-ref of="% averaged"() -> (w506:refnum<vi>)
              n256 = control-ref of="Acquisition cycle"() -> (w505:refnum<vi>)
              n257 = control-ref of="Cancel\nacquisition"() -> (w500:refnum<vi>)
              n258 = local read "Toggle position"() -> (w510:i32)
              n259 = control-ref of="Binned interferogram"() -> (w507:refnum<vi>)
              n260 = Equal?(x=w510, y=1) -> (x = y?=w490:bool)
              n261 = case shown="True" w490 {
                tunnel: ["Sample: physical channels (inputV, ScanDelay X)" "Bright beam: physical channels (inputV, ScanDelay X)"] -> w495
                tunnel: [w519 w521] -> w494
                frame False {
                  n262 = local read "Sample: alignment delay"() -> (w519:i32)
                }
                frame True {
                  n263 = local read "Bright beam: alignment delay"() -> (w521:i32)
                }
              }
              n264 = And(x="Optimize\ninterferogram\nalignment", y="Update alignment") -> (x .and. y?=w491:bool)
              n265 = case shown="True" w490 {
                tunnel: ["Cyc. / intfg.\n(sample)" "Cyc. per intfg. (BB)"] -> w489
                frame False {
                }
                frame True {
                }
              }
              n266 = call "ScanDelay_FTIR_GetSpectrum_Aligning.vi"("Cancel? External"=w500, "% averaged (external)"=w506, "Binned interferogram (external)"=w507, "Python refnum in"=w508, "Optimize\ninterferogram\ndelay"="Optimize\ninterferogram\nalignment", "Acquisition cycle (external)"=w505, "Gain"=1.0, "Displacement\n calibration  factor"="Delay calibratior\nfactor (ps/V)", "Channels to read (input V, ScanDelay)"=w495, "Acquisitions per interferogram"=w489, "Time per\nacquisition (s)"="Time per\nacquisition (s)", "Sampling rate"="Sampling rate", "Delay estimation (pts)"=w494) -> ("Output spectrum"=w501:dbl[][], "Best delay"=w496:i32)  [unwired: 1 in]
              n267 = case shown="True" w491 {
                tunnel: w496 -> [_ w516]
                tunnel: w490 -> [_ w515]
                frame False {
                }
                frame True {
                  # "Update our optimal delay only if we are actively optimizing"
                  n268 = case shown="True" w515 {
                    tunnel: w516 -> [w517 w518]
                    frame False {
                      n269 = local write "Sample: alignment delay"(w517) -> ()
                    }
                    frame True {
                      n270 = local write "Bright beam: alignment delay"(w518) -> ()
                    }
                  }
                }
              }
              n271 = case shown="False" w490 {
                tunnel: [Control_GetSpectrum_LineScanSpectroscopy."Accumulate sample spectrum" Control_GetSpectrum_LineScanSpectroscopy."Accumulate BB spectrum"] -> w499
                tunnel: w501 -> [_ _]
                tunnel: [w525 w530] -> w497
                frame False {
                  n272 = local read "Cancel\nacquisition"() -> (w526:bool)
                  n273 = local read "Halt program"() -> (w527:bool)
                  n274 = Or(x=w526, y=w527) -> (x .or. y?=w525:bool)
                  n275 = local write "Acquisition status"("Accumulating sample spectrum...") -> ()
                }
                frame True {
                  n276 = local read "Cancel\nacquisition"() -> (w532:bool)
                  n277 = local read "Halt program"() -> (w531:bool)
                  n278 = Or(x=w532, y=w531) -> (x .or. y?=w530:bool)
                  n279 = local write "Acquisition status"("Accumulating bright beam spectrum...") -> ()
                }
              }
              n280 = case shown="False" w497 {
                tunnel: w499 -> [w523 _]
                tunnel: [w523 Control_GetSpectrum_LineScanSpectroscopy."Done"] -> w498
                frame False {
                }
                frame True {
                }
              }
            }
            frame "Accumulate BB spectrum" {
              n281 = Empty Array?(array=w536) -> (empty?=w535:bool)
              n282 = case shown="False" w535 {
                tunnel: w548 -> [w563 w565]
                tunnel: w536 -> [w564 _]
                tunnel: [w562 w565] -> w553
                frame False {
                  n283 = Build Array (concatenate)(w564, w563) -> (w562:dbl[][])
                }
                frame True {
                }
              }
              n284 = local read "Apply spectral\nenvelope"() -> (w545:bool)
              n285 = local read "Python scandelay path"() -> (w554:path)
              n286 = local read "Envelope width"() -> (w544:dbl)
              n287 = node(w557, w554, "accumulate_spectra", w556, w553, w553, w545, w544) -> (w555:refnum<k35>, w547:errorcluster, w546:dbl[][])  [unwired: 3 in, 2 out]
              n288 = Index Array(array=w546, index (row) #1=0, index (row) #2=1) -> (element #1=w550:dbl[], element #2=w549:dbl[])  [unwired: 2 in]
              n289 = Bundle("Output spectrum"=w550, "Output spectrum"=w549) -> (→"Accumulated spectrum (amplitude)":T1)  [unwired: 1 in]
              n290 = local write "Python error: spectrum acquisition"(w547) -> ()
              n291 = Not(x="Flip anyway") -> (.not. x?=w541:bool)
              n292 = And(x="Acquire only\nBB 100% curve", y=w541) -> (x .and. y?=w540:bool)
              n293 = case shown="False" w540 {
                tunnel: [Control_GetSpectrum_LineScanSpectroscopy."Flip out BB" Control_GetSpectrum_LineScanSpectroscopy."Attenuate alpha"] -> w543
                frame False {
                }
                frame True {
                  n294 = local write "Toggle position"(2) -> ()
                }
              }
            }
            frame "Flip out BB" {
              n295 = flat-sequence {
                tunnel: w567 -> [w575]
                tunnel: w567 -> [w581]
                frame #0 {
                  n296 = local write "Acquisition status"("Toggling to sample beam ...") -> ()
                }
                frame #1 {
                  n297 = local write "Toggle position"(2) -> ()
                  n298 = call "NewportFlipper.vi"("Settle time (ms)"=w575, "Up/Down"=FALSE) -> ()  [unwired: 10 in]
                }
                frame #2 {
                  w577 = "Returning to bright beam..."
                  n299 = local read "Acquire only\nBB 100% curve"() -> (w580:bool)
                  n300 = local read "Flip anyway"() -> (w579:bool)
                  n301 = local write "Acquisition status"(w577) -> ()
                  n302 = And(x=w580, y=w579) -> (x .and. y?=w578:bool)
                  n303 = case shown="True" w578 {
                    tunnel: w581 -> [_ w582]
                    tunnel: w577 -> [_ _]
                    frame False {
                    }
                    frame True {
                      n304 = call "NewportFlipper.vi"("Settle time (ms)"=w582, "Up/Down"=TRUE) -> ()  [unwired: 10 in]
                    }
                  }
                }
                frame #3 {
                  n305 = local write "Acquisition status"("Acquiring sample beam spectrum...") -> ()
                }
              }
            }
            frame "Accumulate sample spectrum" {
              # "We could now say \"BB-reference\" using \"current point\" whose entry we just populated"
              # "Store data at this point for this accumulation"
              # "Flatten these N spectra from 3 to 2 dimensions"
              # "Finally initialize data holder for sample spectra at all accumulations and all points:\nN accum. x N points x (N freqs x 5)"
              # "2D array of all accumulations at this point\n(from 0 to (# accum+1) )"
              n306 = Empty Array?(array=w596) -> (empty?=w597:bool)
              n307 = case shown="True" w597 {
                tunnel: [w623 w624] -> w592
                tunnel: w596 -> [w623 _]
                tunnel: w591 -> [_ w628]
                frame False {
                }
                frame True {
                  n308 = local read "# of Accumulations"() -> (w627:i32)
                  n309 = for {
                    N: w627 -> [_]
                    tunnel: w628 -> [w631]
                    tunnel: [w629] -> w625 mode=indexing
                    n310 = local read "# of spatial points"() -> (w630:i32)
                    n311 = for {
                      N: w630 -> [_]
                      tunnel: w631 -> [w632]
                      tunnel: [w632] -> w629 mode=indexing
                    }
                  }
                  n312 = Multiply(x=w625, y=0) -> (x*y=w624:dbl[][][][])
                }
              }
              n313 = flat-sequence {
                tunnel: [w619] -> w593
                tunnel: w592 -> [w618]
                tunnel: w591 -> [w617]
                tunnel: [w616] -> w586
                tunnel: [w615] -> w590
                frame #0 {
                  n314 = local read "Current point\nindex"() -> (w616:i32)
                  n315 = local read "# Accumulated"() -> (w615:i32)
                  n316 = local write "Data needed at new point"(FALSE) -> ()
                  n317 = Replace Array Subset(array=w618, new element=w617, index (dim 0)=w615, index (dim 1)=w616) -> (w619:dbl[][][][])  [unwired: 2 in]
                }
              }
              n318 = Index Array(array=w593, index (dim 1)=w586) -> (element=w594:dbl[][][])  [unwired: 3 in]
              n319 = Increment(x=w590) -> (x+1=w587:i32)
              n320 = Array Subset(array=w594, index (dim 0)=0, length (dim 0)=w587) -> (w589:dbl[][][])  [unwired: 4 in]
              n321 = for {
                tunnel: w589 -> [w622] mode=indexing
                shift-right: [w621] -> w588
                shift-left: dbl[][] [] -> [w620]
                n322 = Build Array (concatenate)(w622, w620) -> (w621:dbl[][])
              }
              n323 = local read "Apply spectral\nenvelope"() -> (w600:bool)
              n324 = local read "Python scandelay path"() -> (w609:path)
              n325 = local read "Envelope width"() -> (w599:dbl)
              n326 = node(w612, w609, "accumulate_spectra", w611, w588, w588, w600, w599) -> (w610:refnum<k35>, w603:errorcluster, w601:dbl[][])  [unwired: 3 in, 2 out]
              n327 = local write "Python error: spectrum acquisition"(w603) -> ()
              n328 = Index Array(array=w601, index (row) #1=0, index (row) #2=1) -> (element #1=w606:dbl[], element #2=w605:dbl[])  [unwired: 2 in]
              n329 = Bundle(w606, w605) -> (w598:cluster{dbl[], dbl[]})  [unwired: 1 in]
              n330 = property on="Accumulated spectrum (amplitude)" class="XYGraph (strict)"("Value"=w598) -> ()  [unwired: 2 in, 2 out]
            }
            frame "Await next point" {
              n331 = flat-sequence {
                tunnel: [w647] -> w634
                tunnel: w634 -> [w658]
                tunnel: [w657] -> w633
                tunnel: [w668] -> w635
                tunnel: w633 -> [w665]
                frame #0 {
                  # "Evaluates to true if there are no more spatial points remaining"
                  n332 = local read "Current point\nindex"() -> (w649:i32)
                  n333 = local write "Acquisition status"("Awaiting motion to next point...") -> ()
                  n334 = local read "# of Accumulations"() -> (w654:i32)
                  n335 = local read "# of spatial points"() -> (w651:i32)
                  n336 = local read "# Accumulated"() -> (w648:i32)
                  n337 = Increment(x=w649) -> (x+1=w650:i32)
                  n338 = Increment(x=w648) -> (x+1=w655:i32)
                  n339 = Greater Or Equal?(x=w650, y=w651) -> (x >= y?=w653:bool)
                  n340 = Greater Or Equal?(x=w655, y=w654) -> (x >= y?=w652:bool)
                  n341 = And(x=w653, y=w652) -> (x .and. y?=w647:bool)
                }
                frame #1 {
                  n342 = while {
                    tunnel: w658 -> [w659]
                    tunnel: [w659] -> w657
                    stop <- w660 stop-if-true
                    n343 = local read "Data needed at new point"() -> (w662:bool)
                    n344 = Wait (ms)(milliseconds to wait=5) -> ()  [unwired: 1 out]
                    n345 = local read "Halt program"() -> (w663:bool)
                    n346 = Or(x=w662, y=w663) -> (x .or. y?=w661:bool)
                    n347 = Or(x=w659, y=w661) -> (x .or. y?=w660:bool)
                  }
                }
                frame #2 {
                  n348 = local read "Line done"() -> (w666:bool)
                  n349 = Or(x=w665, y=w666) -> (x .or. y?=w667:bool)
                  n350 = case shown="True" w667 {
                    tunnel: [Control_GetSpectrum_LineScanSpectroscopy."Get Spectrum" Control_GetSpectrum_LineScanSpectroscopy."Assess accumulation"] -> w668
                    frame False {
                      n351 = local write "Acquisition status"("Acquiring sample spectrum...") -> ()
                    }
                    frame True {
                    }
                  }
                }
              }
              n352 = flat-sequence {
                tunnel: [w643] -> w636
                tunnel: w635 -> [w642]
                frame #0 {
                  n353 = local read "Halt program"() -> (w644:bool)
                  n354 = case shown="True" w644 {
                    tunnel: [w645 Control_GetSpectrum_LineScanSpectroscopy."Done"] -> w643
                    tunnel: w642 -> [w645 _]
                    frame False {
                    }
                    frame True {
                    }
                  }
                }
              }
            }
            frame "Assess accumulation" {
              n355 = flat-sequence {
                tunnel: w673 -> [w681]
                tunnel: w672 -> [w680]
                tunnel: [w687] -> w675
                frame #0 {
                  # "Increment accumulation #"
                  n356 = local write "Sample BB Spectra"(w681) -> ()
                  n357 = local write "Sample Spectra at all accumulations"(w680) -> ()
                  n358 = local read "# Accumulated"() -> (w679:i32)
                  n359 = Increment(x=w679) -> (x+1=w678:i32)
                  n360 = local write "# Accumulated"(w678) -> ()
                }
                frame #1 {
                  # "Completion of line signaled us to get here,\nso now we have moved to new line and we should re-set it"
                  n361 = local read "# Accumulated"() -> (w682:i32)
                  n362 = local read "# of Accumulations"() -> (w684:i32)
                  n363 = property on="BB-reference spectrum" class="Bool (strict)"("Val(Sgnl)"=FALSE) -> ()  [unwired: 2 in, 2 out]
                  n364 = local write "Line done"(FALSE) -> ()
                  n365 = Less Or Equal?(x=w684, y=w682) -> (x <= y?=w685:bool)
                  n366 = case shown="True" w685 {
                    tunnel: [w688 Control_GetSpectrum_LineScanSpectroscopy."Finalize"] -> w687
                    frame False {
                      n367 = local read "Replicate\nalpha on\naccumulation"() -> (w689:bool)
                      n368 = case shown="True" w689 {
                        tunnel: [Control_GetSpectrum_LineScanSpectroscopy."Flip in BB" Control_GetSpectrum_LineScanSpectroscopy."Replicate alpha"] -> w688
                        frame False {
                          n369 = local write "Acquisition status"("Toggling to bright beam") -> ()
                        }
                        frame True {
                          n370 = local write "Acquisition status"("Replicating alpha...") -> ()
                        }
                      }
                    }
                    frame True {
                    }
                  }
                }
              }
            }
            frame "Finalize" {
              n371 = local write "Spectrum stored"(TRUE) -> ()
            }
            frame "Done" {
              w703 = FALSE
              n372 = local write "Acquire spectrum"(w703) -> ()
              n373 = local write "Cancel\nacquisition"(w703) -> ()
            }
          }
          n374 = Wait (ms)(milliseconds to wait=5) -> ()  [unwired: 1 out]
        }
      }
      event Timeout {
        n375 = event-data() -> ()  [unwired: 1 in, 3 out]
        n376 = Wait (ms)(milliseconds to wait=w711) -> ()  [unwired: 1 out]
      }
    }
    n377 = Wait (ms)(milliseconds to wait=5) -> ()  [unwired: 1 out]
    n378 = local read "Halt program"() -> (w352:bool)
    "Acquisition status" <- "Ready to acquire spectrum"
  }
  n379 = while {
    stop <- w713 stop-if-true
    w712 = 5
    n380 = Wait (ms)(milliseconds to wait=w712) -> ()  [unwired: 1 out]
    n381 = event shown="[1] \"Next Point\": Value Change" {
      selector: _ -> [_ _]
      dyn-events: _ -> [_ _]
      timeout: w712 -> [_ _]
      event Timeout {
        n382 = event-data() -> ()  [unwired: 1 in, 3 out]
      }
      event "Next Point": Value Change {
        n383 = event-data() -> ("NewVal"=w714:bool)  [unwired: 1 in, 1 out]
        n384 = case shown="True" w714 {
          frame False {
          }
          frame True {
            # "This step \"releases\" update of the point"
            n385 = local read "Current point\nindex"() -> (w718:i32)
            n386 = Decrement(x="# of spatial points") -> (x-1=w716:i32)
            n387 = Less?(x=w718, y=w716) -> (x < y?=w719:bool)
            n388 = case shown="True" w719 {
              tunnel: w718 -> [_ w725]
              tunnel: [0 w724] -> w717
              frame False {
                "Line done" <- TRUE
              }
              frame True {
                n389 = Increment(x=w725) -> (x+1=w724:i32)
              }
            }
            n390 = flat-sequence {
              tunnel: w717 -> [w721]
              frame #0 {
                "Current point\nindex" <- w721
                "Data needed at new point" <- TRUE
              }
            }
          }
        }
      }
    }
    n391 = local read "Halt program"() -> (w713:bool)
  }
  n392 = Close Python Session(session in=w13, error in=w12) -> (11:w9:errorcluster)
  n393 = local write "Python error: activity loop"(w9) -> ()
  n394 = Close Python Session(session in=w3, error in=w2) -> ()  [unwired: 1 out]
